vi "Memory.Array.Get Pointer.vi"(8 "error in (no error)":errorcluster, 11 "Array in":refnum<class "Memory.Array.Void.lvclass">) -> (0 "error out":errorcluster, 2 "Pointer":refnum<class "Memory.Pointer.Void.lvclass">, 3 "Array out":refnum<class "Memory.Array.Void.lvclass">)   [LabVIEW 2016, in "LabVIEW Memory Manager.lvlib" / "Memory.Array.Void.lvclass"]
uses:
  Memory.Array.Void.lvclass
  Pointer/Pointer.Void/Memory.Pointer.Void.lvclass
  Memory.Array.Void.lvclass/Memory.Array.Void.ctl
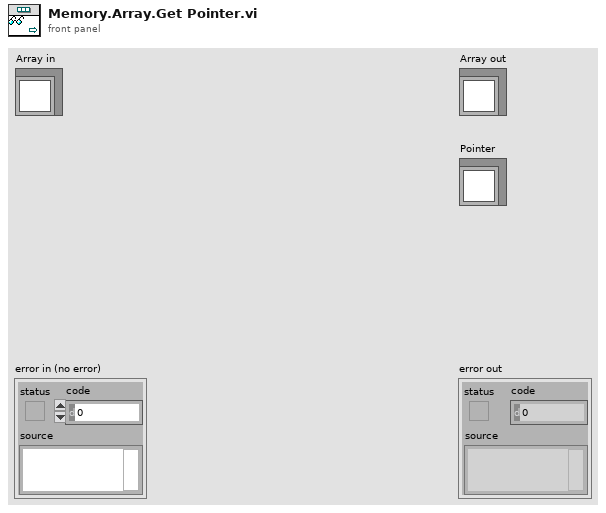
[diagram p1: front panel]
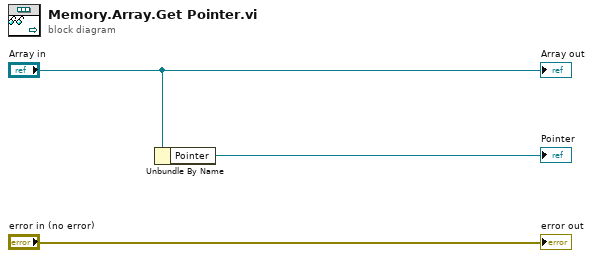
[diagram p0: block diagram]
diagram:
  n1 = Unbundle By Name("Array in") -> ("Pointer"=→"Pointer":refnum<class "Memory.Pointer.Void.lvclass">)
  "error out" <- "error in (no error)"
  "Array out" <- "Array in"
